vi "AddNicknames.vi"(8 "Values":dbl[](array[numeric]), 9 "Nicknames":string[](array[string]), 10 "Base Name":string) -> (1 "Base Name + Nicknames and Values":string)   [LabVIEW 2016]
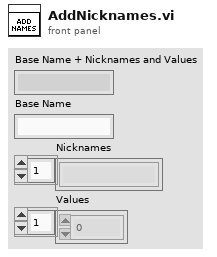
[diagram p1: front panel]
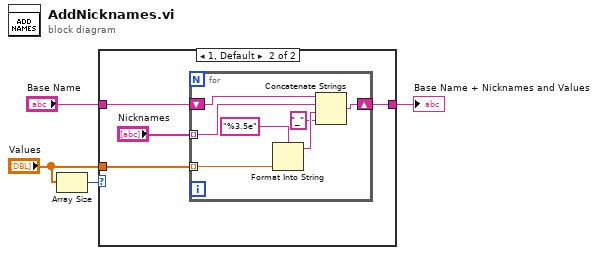
[diagram p0: block diagram]
diagram:
  n1 = Array Size(array="Values") -> (size(s)=w2:i32)
  n2 = case shown="1, Default" w2 {
    tunnel: "Base Name" -> [w5 w8]
    tunnel: [w5 w7] -> w3
    tunnel: "Values" -> [_ w6]
    frame 0 {
    }
    frame 1, Default {
      n3 = for {
        shift-right: [w16] -> w7
        shift-left: w8 -> [w15]
        tunnel: "Nicknames" -> [w14] mode=indexing
        tunnel: w6 -> [w13] mode=indexing
        n4 = Format Into String(format string="%3.5e", w13) -> (resulting string=w11:string)  [unwired: 2 in, 1 out]
        n5 = Concatenate Strings(w15, w14, w11, "_" ("string")) -> (w16:string)
      }
    }
  }
  "Base Name + Nicknames and Values" <- w3
